vi "Get Digital Pattern.vi"(8 "error in (no error)":errorcluster, 11 "Item Ref in":T1 format="%.0x") -> (0 "error out":errorcluster, 2 "EPT Pattern":T2, 3 "Item Ref out":T1 format="%.0x")   [LabVIEW 2019, in "Engine Simulation Toolkit System Explorer.lvlib"]
uses:
  Engine Simulation Toolkit System Explorer.lvlib
  <vilib>/NI VeriStand/Custom Device API/Custom Device Item Ref.ctl
  Digital Pattern.ctl
  Digital Pattern Base.ctl
  Digital Pattern Remove Edge.ctl
  Digital Pattern Add Pulse.ctl
  Shared/Properties.vi
  <vilib>/NI VeriStand/Custom Device API/Get Item Property (Double).vi
  <vilib>/NI VeriStand/Custom Device API/Get Item Property (U16).vi
  <vilib>/NI VeriStand/Custom Device API/Get Item Property (String).vi
  <vilib>/NI VeriStand/Custom Device API/Get Item Property (Boolean).vi
  <vilib>/NI VeriStand/Custom Device API/Custom Device API.lvlib
  Shared/Engine Simulation Toolkit Shared.lvlib
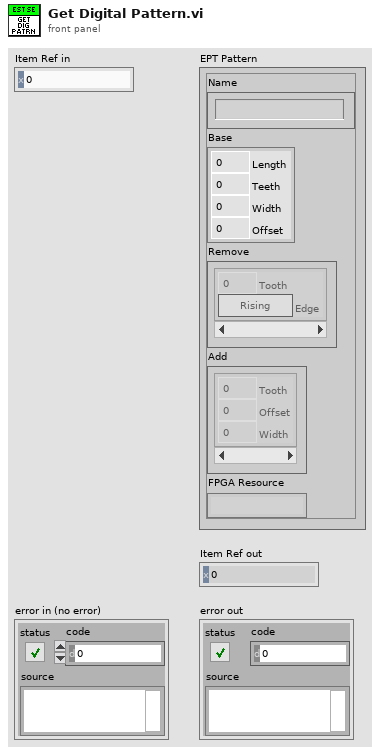
[diagram p1: front panel]
types:
  T1 = typedef "Custom Device API.lvlib/Custom Device Item Ref.ctl" = u64
  T2 = typedef "Engine Simulation Toolkit System Explorer.lvlib/Digital Pattern.ctl" = cluster{"Name":string, "Base":T3, "Remove":T4[], "Add":T5[], "FPGA Resource":string}
  T3 = typedef "Engine Simulation Toolkit System Explorer.lvlib/Digital Pattern Base.ctl" = cluster{"Length":dbl, "Teeth":u16, "Width":dbl, "Offset":dbl}
  T4 = typedef "Engine Simulation Toolkit System Explorer.lvlib/Digital Pattern Remove Edge.ctl" = cluster{"Tooth":u16, "Edge":bool}
  T5 = typedef "Engine Simulation Toolkit System Explorer.lvlib/Digital Pattern Add Pulse.ctl" = cluster{"Tooth":u16, "Offset":dbl, "Width":dbl}
  T6 = typedef "Custom Device API.lvlib/Custom Device Item Info.ctl" = cluster{"Name":string, "Is Channel":bool, "GUID":string, "Is Waveform":bool}
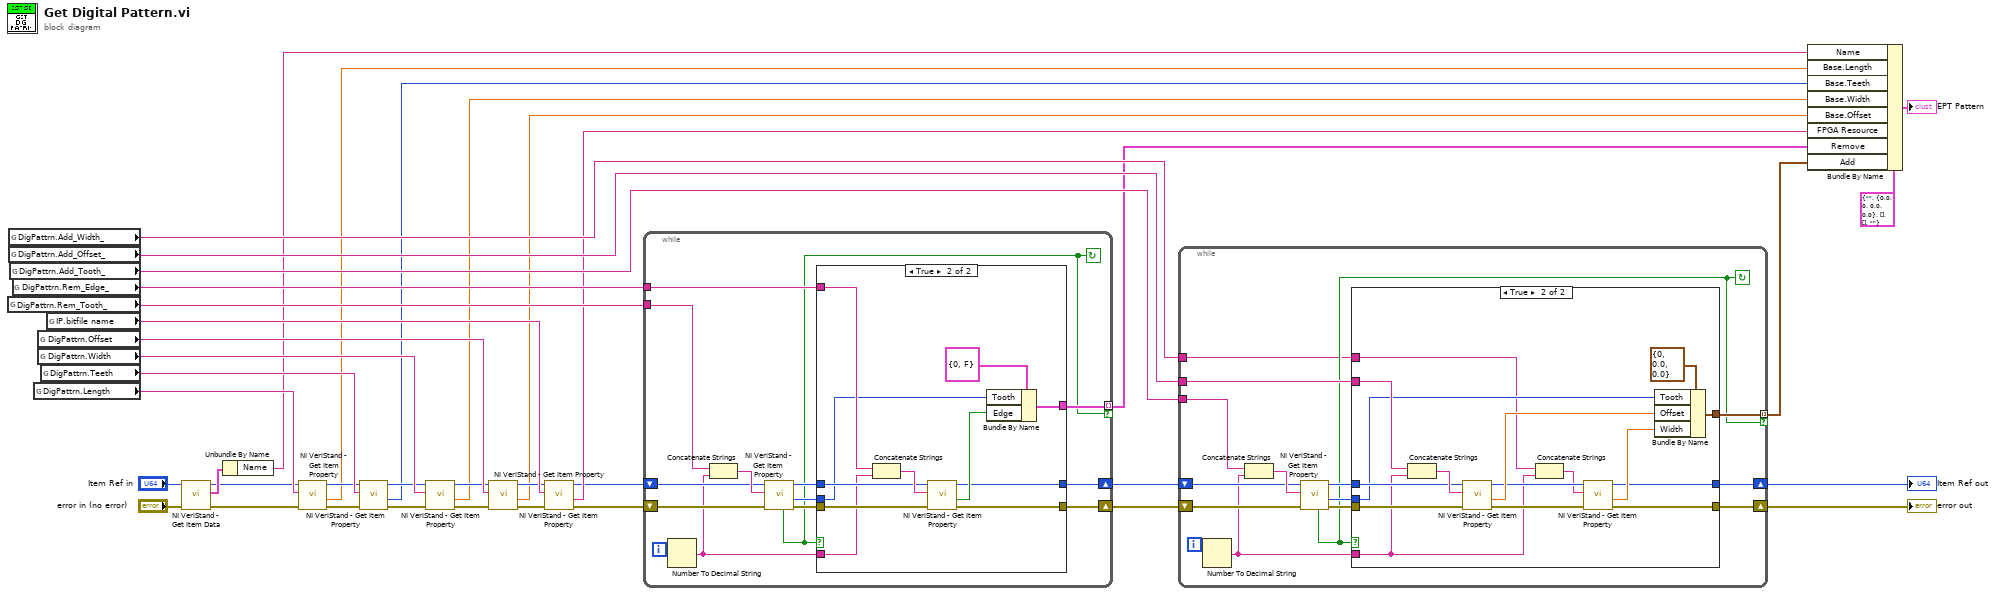
[diagram p0: block diagram]
diagram:
  n1 = global read "Properties.vi" "DigPattrn.Rem_Tooth_"() -> (w35:string)
  n2 = global read "Properties.vi" "DigPattrn.Add_Width_"() -> (w39:string)
  n3 = global read "Properties.vi" "DigPattrn.Add_Offset_"() -> (w38:string)
  n4 = global read "Properties.vi" "DigPattrn.Add_Tooth_"() -> (w37:string)
  n5 = global read "Properties.vi" "DigPattrn.Rem_Edge_"() -> (w36:string)
  n6 = global read "Properties.vi" "DigPattrn.Length"() -> (w30:string)
  n7 = global read "Properties.vi" "DigPattrn.Offset"() -> (w33:string)
  n8 = global read "Properties.vi" "DigPattrn.Width"() -> (w32:string)
  n9 = global read "Properties.vi" "DigPattrn.Teeth"() -> (w31:string)
  n10 = global read "Properties.vi" "IP.bitfile name"() -> (w34:string)
  n11 = call <vilib>:"NI VeriStand - Get Item Data.vi"("error in (no error)"="error in (no error)", "Item Ref in"="Item Ref in") -> ("error out"=w3:errorcluster, "Item Info"=w6:T6, "Item Ref out"=w4:T1)  [unwired: 6 in, 1 out]
  n12 = Unbundle By Name(w6) -> ("Name"=w28:string)
  n13 = call-poly <vilib>:"NI VeriStand - Get Item Property.vi"("error in (no error)"=w3, "Property Name"=w30, "Item Ref in"=w4) -> ("error out"=w11:errorcluster, "Value"=w9:dbl, "Item Ref out"=w10:T1)  [unwired: 5 in, 1 out]
  n14 = call-poly <vilib>:"NI VeriStand - Get Item Property.vi"("error in (no error)"=w11, "Property Name"=w31, "Item Ref in"=w10) -> ("error out"=w14:errorcluster, "Value"=w12:u16, "Item Ref out"=w13:T1)  [unwired: 5 in, 1 out]
  n15 = call-poly <vilib>:"NI VeriStand - Get Item Property.vi"("error in (no error)"=w14, "Property Name"=w32, "Item Ref in"=w13) -> ("error out"=w17:errorcluster, "Value"=w15:dbl, "Item Ref out"=w16:T1)  [unwired: 5 in, 1 out]
  n16 = call-poly <vilib>:"NI VeriStand - Get Item Property.vi"("error in (no error)"=w17, "Property Name"=w33, "Item Ref in"=w16) -> ("error out"=w26:errorcluster, "Value"=w18:dbl, "Item Ref out"=w25:T1)  [unwired: 5 in, 1 out]
  n17 = call-poly <vilib>:"NI VeriStand - Get Item Property.vi"("error in (no error)"=w26, "Property Name"=w34, "Item Ref in"=w25) -> ("error out"=w23:errorcluster, "Value"=w27:string, "Item Ref out"=w24:T1)  [unwired: 5 in, 1 out]
  n18 = while {
    shift-right: [w40] -> w21
    shift-left: w23 -> [w51]
    shift-right: [w41] -> w20
    shift-left: w24 -> [w52]
    tunnel: w36 -> [w46]
    tunnel: w35 -> [w44]
    tunnel: [w43] -> w19 mode=indexing if=w42
    i -> [w50]
    stop <- w42 continue-if-true
    n19 = Number To Decimal String(number=w50) -> (decimal integer string=w45:string)  [unwired: 1 in]
    n20 = Concatenate Strings(w44, w45) -> (w53:string)
    n21 = call-poly <vilib>:"NI VeriStand - Get Item Property.vi"("error in (no error)"=w51, "Property Name"=w53, "Item Ref in"=w52) -> ("error out"=w49:errorcluster, "Value"=w47:u16, "Item Ref out"=w48:T1, "Found?"=w42:bool)  [unwired: 5 in]
    n22 = case shown="True" w42 {
      tunnel: w49 -> [w54 w63]
      tunnel: w48 -> [w55 w64]
      tunnel: w47 -> [_ w60]
      tunnel: w46 -> [_ w62]
      tunnel: w45 -> [_ w61]
      tunnel: [w54 w58] -> w40
      tunnel: [w55 w57] -> w41
      tunnel: [_ w56] -> w43
      frame False {
      }
      frame True {
        n23 = Concatenate Strings(w62, w61) -> (w65:string)
        n24 = call-poly <vilib>:"NI VeriStand - Get Item Property.vi"("error in (no error)"=w63, "Property Name"=w65, "Item Ref in"=w64) -> ("error out"=w58:errorcluster, "Value"=w59:bool, "Item Ref out"=w57:T1)  [unwired: 5 in, 1 out]
        n25 = Bundle By Name(cluster=T4 {"Tooth"=0, "Edge"=FALSE} ("Remove Edge"), "Tooth"=w60, "Edge"=w59) -> (w56:T4)
      }
    }
  }
  n26 = while {
    shift-right: [w68] -> w7
    shift-left: w21 -> [w79]
    shift-right: [w69] -> w29
    shift-left: w20 -> [w80]
    tunnel: w38 -> [w74]
    tunnel: w37 -> [w72]
    tunnel: [w71] -> w22 mode=indexing if=w70
    tunnel: w39 -> [w67]
    i -> [w78]
    stop <- w70 continue-if-true
    n27 = Number To Decimal String(number=w78) -> (decimal integer string=w73:string)  [unwired: 1 in]
    n28 = Concatenate Strings(w72, w73) -> (w81:string)
    n29 = call-poly <vilib>:"NI VeriStand - Get Item Property.vi"("error in (no error)"=w79, "Property Name"=w81, "Item Ref in"=w80) -> ("error out"=w77:errorcluster, "Value"=w75:u16, "Item Ref out"=w76:T1, "Found?"=w70:bool)  [unwired: 5 in]
    n30 = case shown="True" w70 {
      tunnel: w77 -> [w82 w96]
      tunnel: w76 -> [w83 w97]
      tunnel: w75 -> [_ w94]
      tunnel: w74 -> [_ w95]
      tunnel: w73 -> [_ w85]
      tunnel: [w82 w89] -> w68
      tunnel: [w83 w87] -> w69
      tunnel: [_ w92] -> w71
      tunnel: w67 -> [_ w86]
      frame False {
      }
      frame True {
        n31 = Concatenate Strings(w95, w85) -> (w98:string)
        n32 = call-poly <vilib>:"NI VeriStand - Get Item Property.vi"("error in (no error)"=w96, "Property Name"=w98, "Item Ref in"=w97) -> ("error out"=w90:errorcluster, "Value"=w93:dbl, "Item Ref out"=w91:T1)  [unwired: 5 in, 1 out]
        n33 = Concatenate Strings(w86, w85) -> (w84:string)
        n34 = call-poly <vilib>:"NI VeriStand - Get Item Property.vi"("error in (no error)"=w90, "Property Name"=w84, "Item Ref in"=w91) -> ("error out"=w89:errorcluster, "Value"=w88:dbl, "Item Ref out"=w87:T1)  [unwired: 5 in, 1 out]
        n35 = Bundle By Name(cluster=T5 {"Tooth"=0, "Offset"=0.0, "Width"=0.0} ("Add Pulse"), "Tooth"=w94, "Offset"=w93, "Width"=w88) -> (w92:T5)
      }
    }
  }
  "Item Ref out" <- w29
  "error out" <- w7
  n36 = Bundle By Name(cluster=T2 {"Name"="", "Base"={"Length"=0.0, "Teeth"=0, "Width"=0.0, "Offset"=0.0}, "Remove"=[], "Add"=[], "FPGA Resource"=""} ("EPT Pattern"), "Name"=w28, "Base.Length"=w9, "Base.Teeth"=w12, "Base.Width"=w15, "Base.Offset"=w18, "FPGA Resource"=w27, "Remove"=w19, "Add"=w22) -> (→"EPT Pattern":T2)
